vi "create daemon exec.vi"(8 "error in (no error)":errorcluster) -> (0 "error out":errorcluster)   [LabVIEW 2016, in "update.lvlib"]
uses:
  update.lvlib
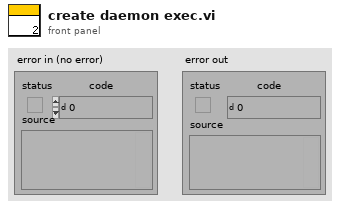
[diagram p1: front panel]
types:
  T1 = enum16{"open", "replace", "create", "open or create", "replace or create", "replace or create with confirmation"}
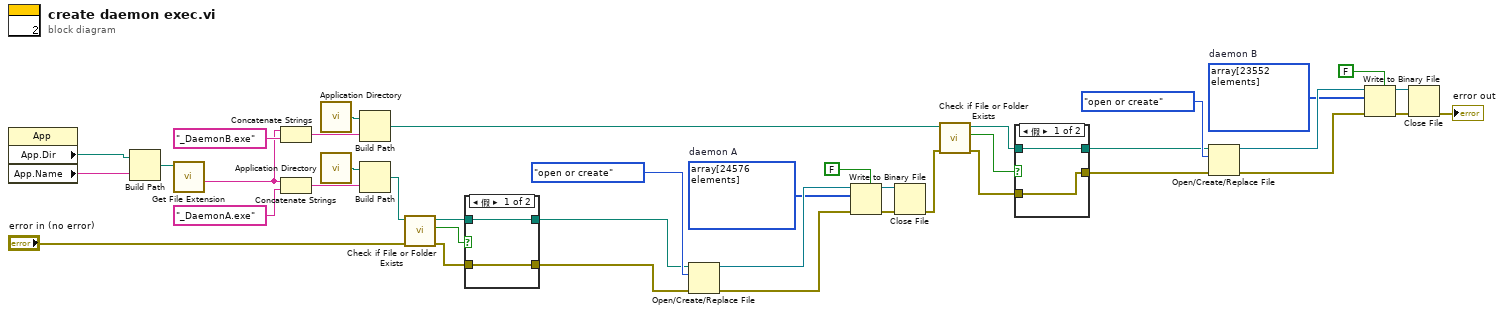
[diagram p0: block diagram]
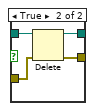
[diagram p2: hidden frame]
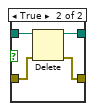
[diagram p3: hidden frame]
diagram:
  w18 = u8[] array[23552 elements]  # daemon B
  w19 = u8[] array[24576 elements]  # daemon A
  n1 = property class="App"() -> ("App.Dir"=w17:path, "App.Name"=w16:string)  [unwired: 2 in, 2 out]
  n2 = Build Path(base path=w17, name or relative path=w16) -> (appended path=w15:path)
  n3 = call <vilib>:"Get File Extension.vi"("file"=w15) -> ("filename without extension"=w22:string)  [unwired: 6 in, 4 out]
  n4 = Concatenate Strings(w22, "_DaemonB.exe" ("名称或相对路径")) -> (w21:string)
  n5 = Concatenate Strings(w22, "_DaemonA.exe" ("名称或相对路径")) -> (w24:string)
  n6 = call <vilib>:"Application Directory.vi"() -> ("Application Directory"=w26:path)
  n7 = call <vilib>:"Application Directory.vi"() -> ("Application Directory"=w39:path)
  n8 = Build Path(base path=w26, name or relative path=w21) -> (appended path=w5:path)
  n9 = Build Path(base path=w39, name or relative path=w24) -> (appended path=w14:path)
  n10 = call <vilib>:"Check if File or Folder Exists.vi"("error in (no error)"="error in (no error)", "path"=w14) -> ("error out"=w11:errorcluster, "file or folder exists?"=w13:bool, "dup path"=w12:path)  [unwired: 7 in]
  n11 = case shown="假" w13 {
    tunnel: w12 -> [w40 w45]
    tunnel: w11 -> [w41 w44]
    tunnel: [w41 w43] -> w6
    tunnel: [w40 w42] -> w2
    frame False {
    }
    frame True {
      n12 = Delete(path (use dialog)=w45, error in=w44) -> (deleted path=w42:path, error out=w43:errorcluster)  [unwired: 3 in, 1 out]
    }
  }
  n13 = Open/Create/Replace File(file path (use dialog)=w2, error in=w6, operation (0:open)=T1."open or create" ("操作(0:open)")) -> (refnum out=w37:refnum<file>, error out=w36:errorcluster)  [unwired: 3 in, 1 out]
  n14 = Write to Binary File(file (use dialog)=w37, data=w19, error in=w36, 5:FALSE ("预置数组或字符串大小？ (T)")) -> (refnum out=w33:refnum<file>, error out=w34:errorcluster)  [unwired: 2 in, 1 out]
  n15 = Close File(refnum=w33, error in=w34) -> (error out=w4:errorcluster)  [unwired: 1 out]
  n16 = call <vilib>:"Check if File or Folder Exists.vi"("error in (no error)"=w4, "path"=w5) -> ("error out"=w10:errorcluster, "file or folder exists?"=w8:bool, "dup path"=w9:path)  [unwired: 7 in]
  n17 = case shown="假" w8 {
    tunnel: w9 -> [w47 w51]
    tunnel: w10 -> [w46 w50]
    tunnel: [w46 w49] -> w3
    tunnel: [w47 w48] -> w1
    frame False {
    }
    frame True {
      n18 = Delete(path (use dialog)=w51, error in=w50) -> (deleted path=w48:path, error out=w49:errorcluster)  [unwired: 3 in, 1 out]
    }
  }
  n19 = Open/Create/Replace File(file path (use dialog)=w1, error in=w3, operation (0:open)=T1."open or create" ("操作(0:open)")) -> (refnum out=w28:refnum<file>, error out=w29:errorcluster)  [unwired: 3 in, 1 out]
  n20 = Write to Binary File(file (use dialog)=w28, data=w18, error in=w29, 5:FALSE ("预置数组或字符串大小？ (T)")) -> (refnum out=w32:refnum<file>, error out=w31:errorcluster)  [unwired: 2 in, 1 out]
  n21 = Close File(refnum=w32, error in=w31) -> (error out=→"error out":errorcluster)  [unwired: 1 out]
